vi "Read Value (by key).vi"(8 "error in (no error)":errorcluster, 10 "key":string, 11 "URI in":refnum<class "URI.lvclass">) -> (0 "error out":errorcluster, 1 "found":bool, 2 "value":string, 3 "URI out":refnum<class "URI.lvclass">)   [LabVIEW 2013, in "openURI.lvlib" / "URI.lvclass"]
uses:
  URI.lvclass
  URI.lvclass/URI.ctl
  components/query/URI-Component.Query.lvclass/URI-Component.Query.ctl
  components/query/URI-Component.Query.lvclass
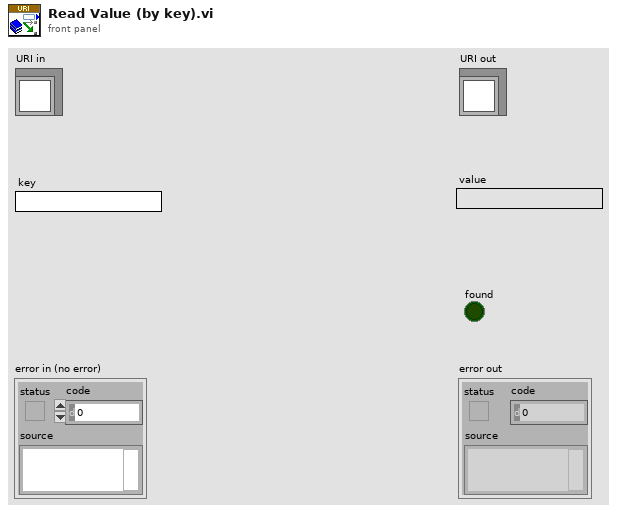
[diagram p1: front panel]
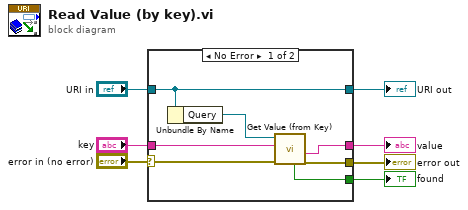
[diagram p0: block diagram]
diagram:
  n1 = case shown="No Error" "error in (no error)" {
    selector: "error in (no error)" -> [w10 w16]
    tunnel: [w9 w16] -> w6
    tunnel: [w14 w15] -> w4
    tunnel: "URI in" -> [w14 w15]
    tunnel: [w11 _] -> w3
    tunnel: "key" -> [w12 _]
    tunnel: [w8 _] -> w1
    frame No Error {
      n2 = Unbundle By Name(w14) -> ("Query"=w13:refnum<class "URI-Component.Query.lvclass">)
      n3 = call "Get Value (from Key).vi"("error in (no error)"=w10, "key"=w12, "URI-Component.Query in"=w13) -> ("error out"=w9:errorcluster, "value"=w11:string, "found"=w8:bool)  [unwired: 4 in, 2 out]
    }
    frame Error {
    }
  }
  "error out" <- w6
  "URI out" <- w4
  "value" <- w3
  "found" <- w1
